vi "Add Weighted Images (ARGB).vi"(5 "B":dbl=0.5, 6 "C (Default: 0)":dbl, 7 "A":dbl=0.5, 8 "error in (no error)":errorcluster, 9 "ARGB Image Destination":T1, 10 "ARGB Image B":T1, 11 "ARGB Image A":T1) -> (0 "error out":errorcluster, 3 "ARGB Image Destination (duplicate)":T1)   [LabVIEW 2020, in "g_ar_toolkit.image.lvlib"]
uses:
  g_ar_toolkit.image.lvlib
  ARGB Image.ctl
  000615f7-9334-4574-8f7b-324cbbba12df.vi
  g_ar_toolkit.common/Module Path.vi
  <vilib>/Utility/error.llb/Error Cluster From Error Code.vi
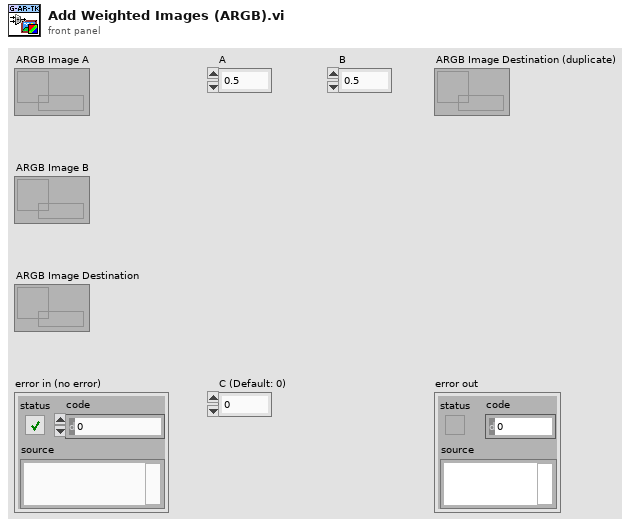
[diagram p1: front panel]
types:
  T1 = typedef "g_ar_toolkit.image.lvlib/ARGB Image.ctl" = refnum<data-value>
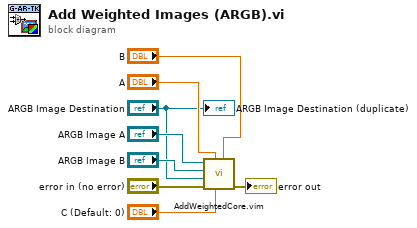
[diagram p0: block diagram]
diagram:
  n1 = call "AddWeightedCore.vim"("B"="B", "C"="C (Default: 0)", "A"="A", "error in (no error)"="error in (no error)", "Dst"="ARGB Image Destination", "Image B"="ARGB Image B", "Image A"="ARGB Image A") -> ("error out"=→"error out":errorcluster)  [unwired: 4 in]
  "ARGB Image Destination (duplicate)" <- "ARGB Image Destination"
